vi "Autonomous Independent V.5.0.vi"() -> ()   [LabVIEW 2016]
doc: "This VI is called when autonomous begins, and will automatically be terminated when autonomous ends. You can carry out timed or sensor driven robot movement independently without needing to return to the caller."
uses:
  <vilib>/Rock Robotics/WPI/Camera/WPI_CameraImageSize.ctl
  <vilib>/Rock Robotics/WPI/ThirdParty/CanMotor/TalonSRX/WPI_CANTalonSRX_BrakeOverride.ctl
  <vilib>/Rock Robotics/WPI/Utilities/WPI_GetSetVariantRefNum.vi
  Robot Global Data V.5.0.vi
  <vilib>/Rock Robotics/Network Tables/NT Read String.vi
panel:
  out "Angle for Gyro":dbl
  out "image size":T1=enum."320x240"
  out "Height":dbl format="%#_13g"
  out "Width":dbl format="%#_13g"
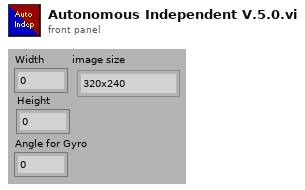
[diagram p1: front panel]
types:
  T1 = typedef "WPI_CameraImageSize.ctl" = enum16{"640x480", "320x240", "160x120", "Custom"}
  T2 = typedef "WPI_CANTalonSRX_BrakeOverride.ctl" = enum8{"No Override", "Override to Coast", "Override to Brake"}
  T3 = cluster{"Distance (ft)":dbl, "Score":dbl, "Normalized":cluster{"Center":cluster{dbl, dbl}, "Rectangle":cluster{"Numeric":dbl, "Numeric 2":dbl, "Numeric 3":dbl, "Numeric 5":dbl}}, "Pixels":cluster{"Center":cluster{dbl, dbl}, "Rectangle":cluster{"Numeric":dbl, "Numeric 2":dbl, "Numeric 3":dbl, "Numeric 5":dbl}}}
  T4 = cluster{"Center":cluster{dbl, dbl}, "Rectangle":cluster{"Numeric":dbl, "Numeric 2":dbl, "Numeric 3":dbl, "Numeric 5":dbl}}
  T5 = cluster{"Numeric":dbl, "Numeric 2":dbl, "Numeric 3":dbl, "Numeric 5":dbl}
  T6 = typedef "WPI_RobotDriveDevRef.ctl" = cluster{"DevStatus":errorcluster, "Motors[]":T7[], "Square Inputs":bool, "Max Output":dbl}
  T7 = typedef "WPI_MotorControlDeviceRef.ctl" = cluster{"DeviceStatus":errorcluster, "Type":T8, "PWM":cluster{"PWM Channel":T9, "DeadBand":T10}, "CAN":cluster{"Device Number":u8, "SetOutput VI Ref":variant, "GetOutput VI Ref":variant, "Enable VI Ref":variant, "Disable VI Ref":variant, "Data":variant}, "Invert":bool}
  T8 = typedef "WPI_MotorControlType.ctl" = enum16{"PWM", "CAN"}
  T9 = typedef "FPGA_DIOPWMChannel.ctl" = enum8{"PWM 0", "PWM 1", "PWM 2", "PWM 3", "PWM 4", "PWM 5", "PWM 6", "PWM 7", "PWM 8", "PWM 9", "PWM MXP 0", "PWM MXP 1", "PWM MXP 2", "PWM MXP 3", "PWM MXP 4", "PWM MXP 5", "PWM MXP 6", "PWM MXP 7", "PWM MXP 8", "PWM MXP 9", "Invalid"}
  T10 = typedef "WPI_PWMDeadband.ctl" = cluster{"Name":string, "maxPositivePwm":i32, "minPositivePwm":i32, "centerPwm":i32, "maxNegativePwm":i32, "minNegativePwm":i32, "angularRange":u16}
  T11 = typedef "WPI_CANTalonSRX_GlobalStatus.ctl" = cluster{"Applied Throttle":dbl, "Module Enabled":bool, "CAN Error":errorcluster, "Closed Loop Error":dbl, "Forward Limit Switch Closed":bool, "Reverse Limit Switch Closed":bool, "Sensor Position":dbl, "Sensor Velocity":dbl, "Current":dbl, "Sticky Fault - Over Temp":bool, "Sticky Fault - Under Voltage":bool, "Sticky Fault - Forward Limit":bool, "Sticky Fault - Reverse Limit":bool, "Sticky Fault - Forward Soft Limit":bool, "Sticky Fault - Reverse Soft Limit":bool, "Brake is Enabled":bool, "Encoder Position":dbl, "Encoder Velocity":dbl, "Encoder Index Count":dbl, "Encoder A Pin State":bool, "Encoder B Pin State":bool, "Encoder Index Pin State":bool, "Analog In":dbl, "Analog In Velocity":dbl, "Temperature (C)":dbl, "Battery Voltage":dbl, "Control 5 Is Supported":bool, "Current Profile Slot Select":dbl, "Pos Div 8":bool, "Vel Div 4":bool, "Pulse Width Position":i32, "Pulse Width Velocity":i32, "Pulse Width Rise To Rise (us)":i32, "Pulse Width Rise To Fall (us)":i32, "Mot Prof Active Is Under Run":bool, "Mot Prof Active Has Under Run":bool, "Mot Prof Active Is Last":bool, "Mot Prof Active Velocity Only":bool, "Mot Prof Active Is Valid":bool, "Mot Prof Buffer Is Full":bool, "Mot Prof Active Profile Slot Select":i32, "Mot Prof NextID":i32, "Mot Prof Count":i32, "Mot Prof Active Velocity":dbl, "Mot Prof Active Position":dbl, "Mot Prof Output Enable":i32}
  T12 = typedef "WPI_GyroDevRef.ctl" = cluster{"DevStatus":errorcluster, "Analog Channel":T13, "Offset":dbl, "Gain (VoltsPerDegree/Second)":dbl, "Gyro Type":enum16{"Analog", "XRS450"}, "Handle":i32, "SPI Bus":T14, "Device Found":bool, "Sample Rate":dbl, "Calibrate On Open":bool}
  T13 = typedef "FPGA_AIChannel.ctl" = enum8{"AI 0", "AI 1", "AI 2", "AI 3", "AI MXP 0", "AI MXP 1", "AI MXP 2", "AI MXP 3", "Invalid"}
  T14 = typedef "spi_bus.ctl" = enum16{"SPI On-Board, CS0", "SPI On-Board, CS1", "SPI On-Board, CS2", "SPI On-Board, CS3", "SPI MXP", "Invalid"}
  T15 = typedef "WPI_ServoDeviceRef.ctl" = cluster{"DeviceStatus":errorcluster, "PWM Channel":T9, "DeadBand":T10}
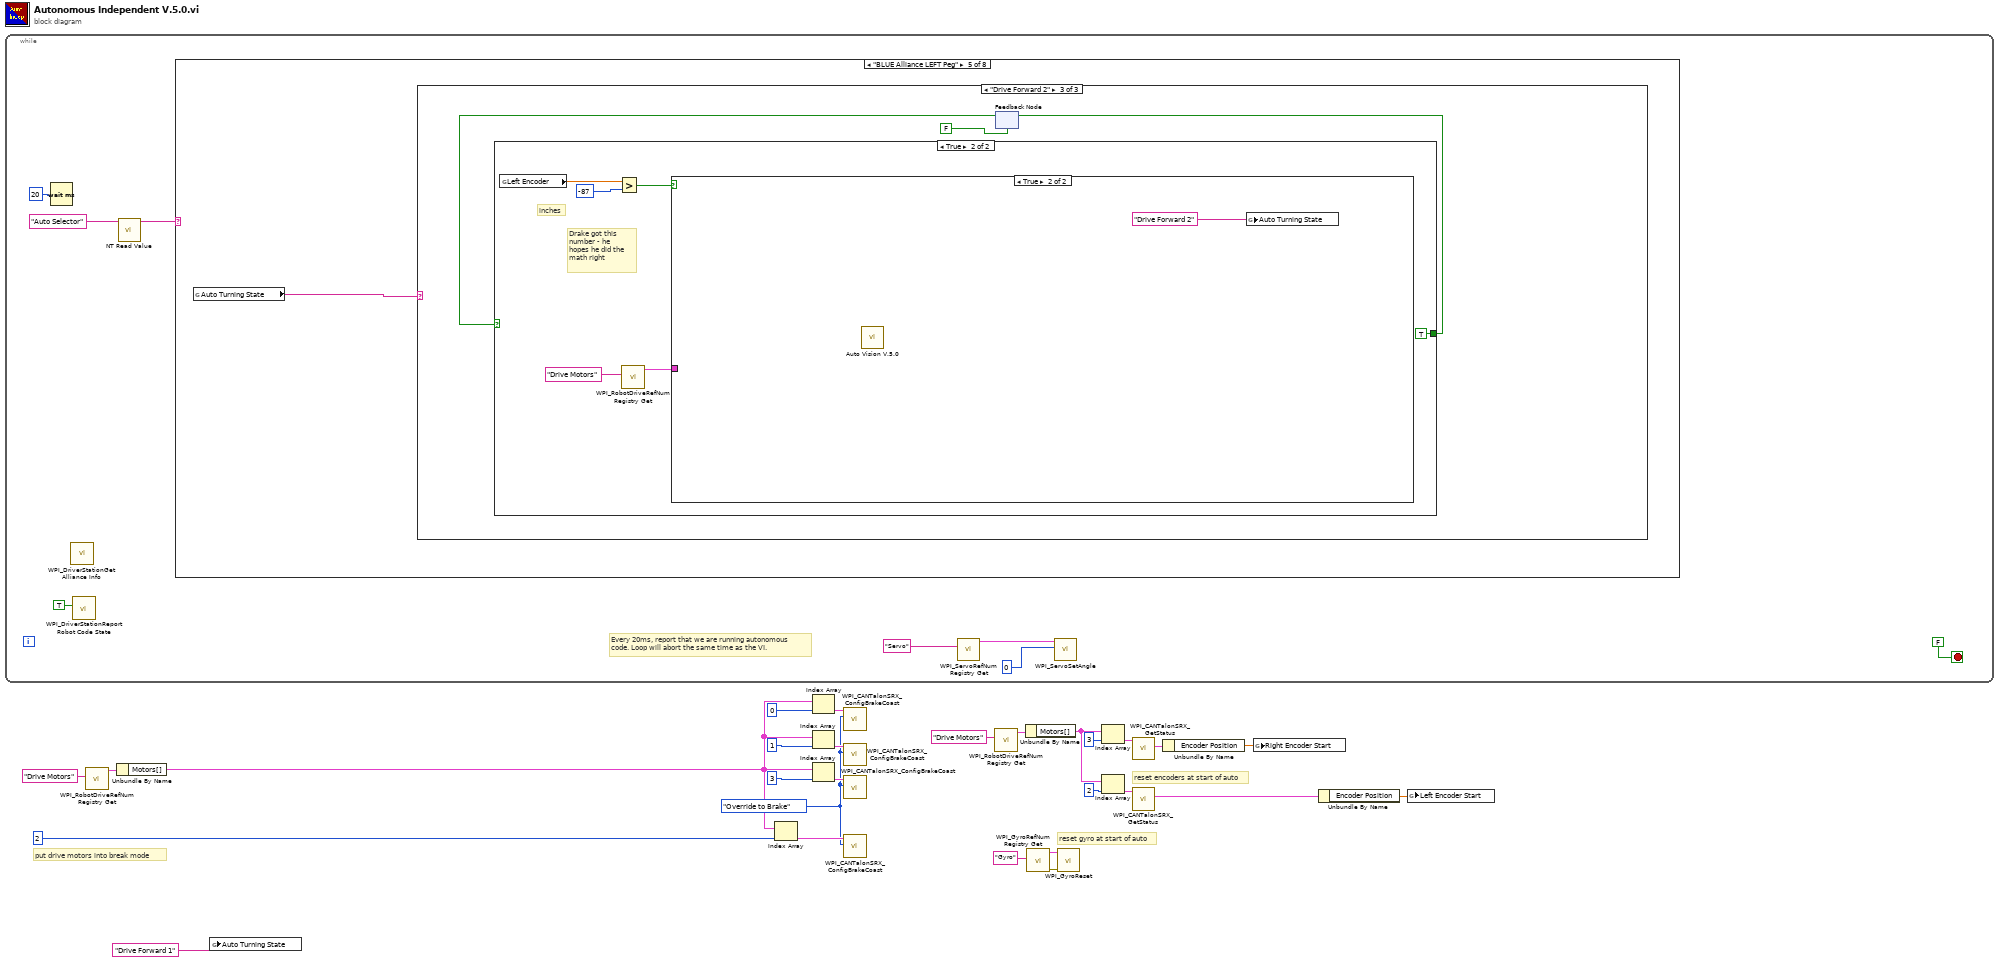
[diagram p0: block diagram]
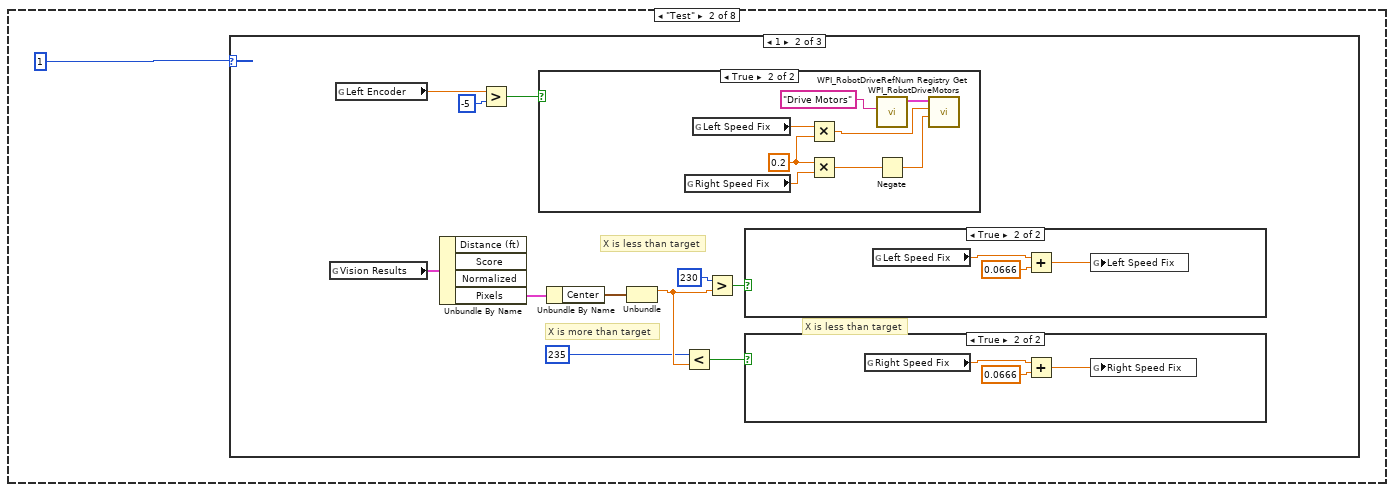
[diagram p3: hidden frame]
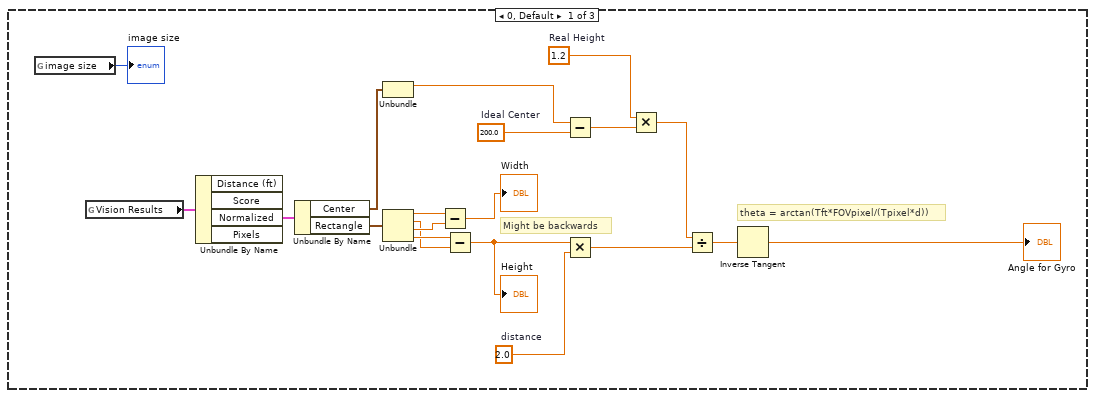
[diagram p4: hidden frame]
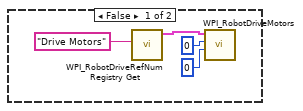
[diagram p5: hidden frame]
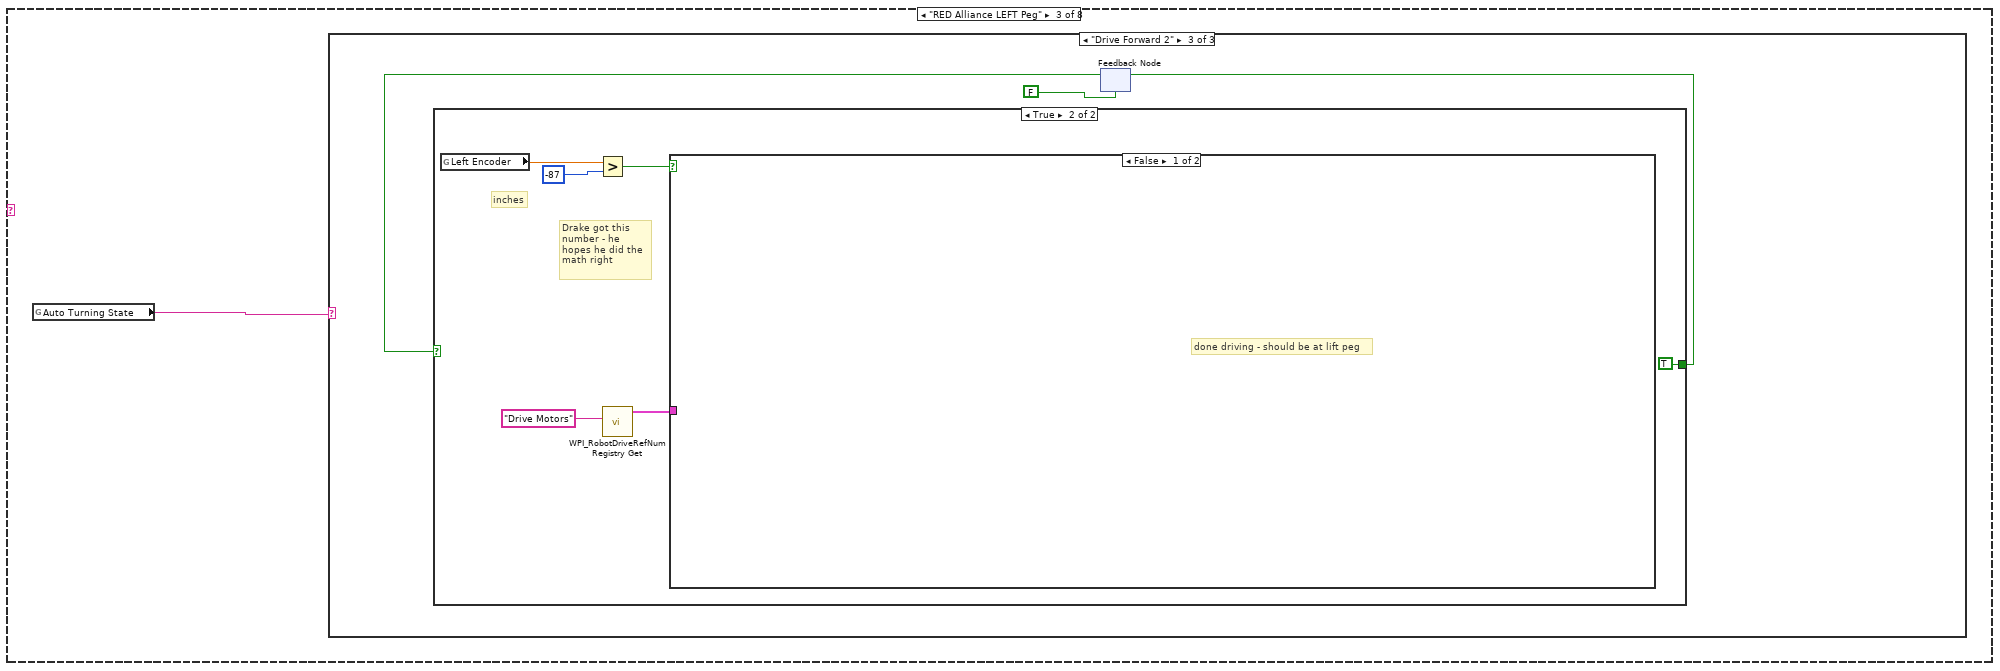
[diagram p9: hidden frame]
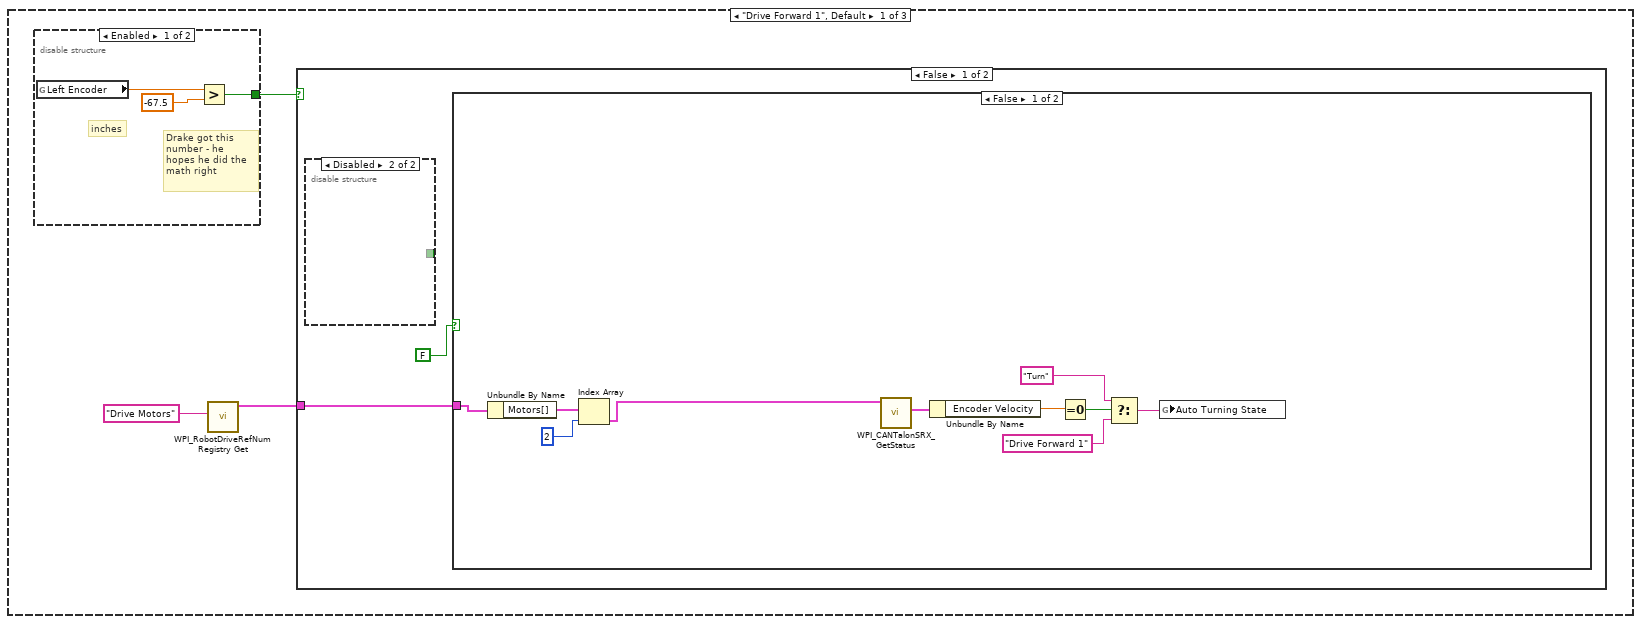
[diagram p10: hidden frame]
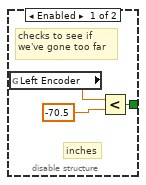
[diagram p12: hidden frame]
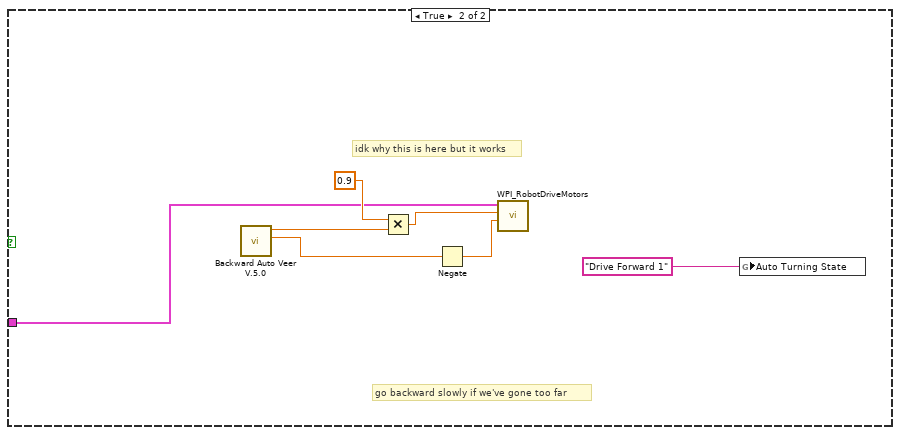
[diagram p13: hidden frame]
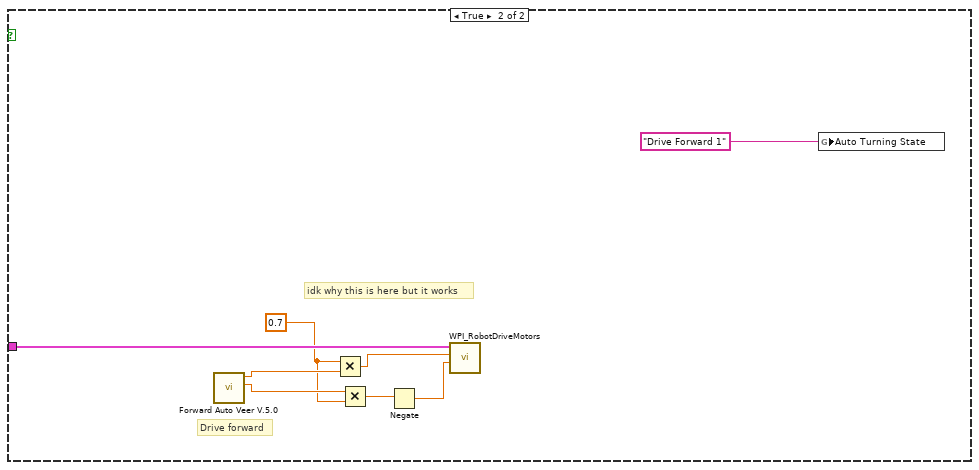
[diagram p14: hidden frame]
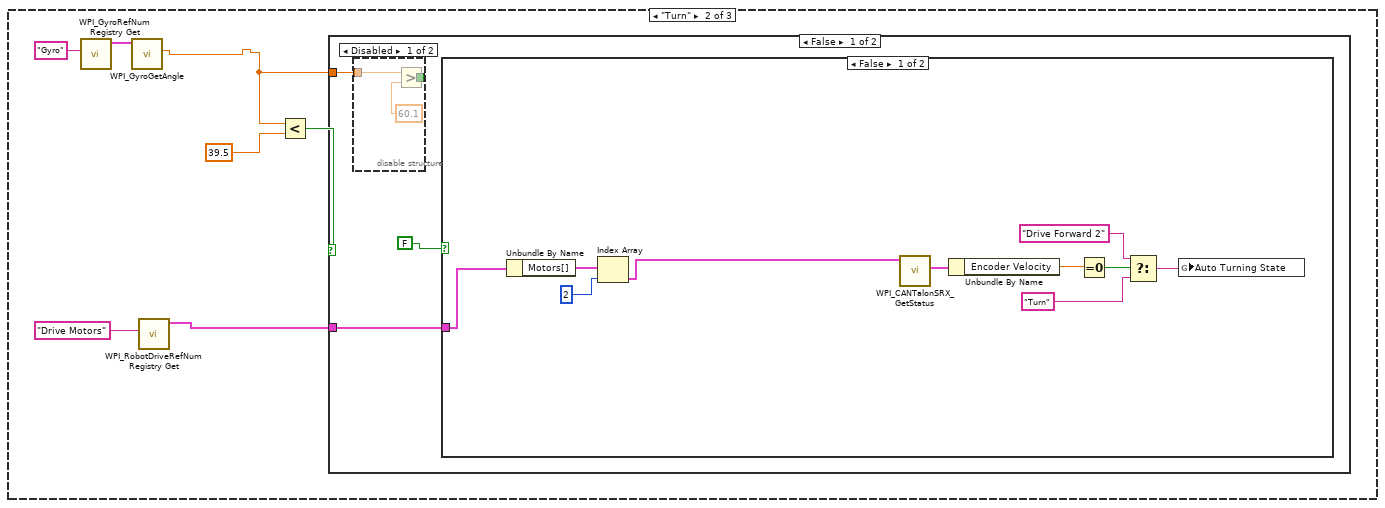
[diagram p15: hidden frame]
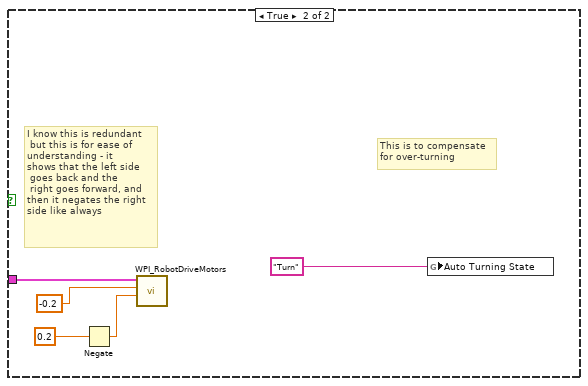
[diagram p17: hidden frame]
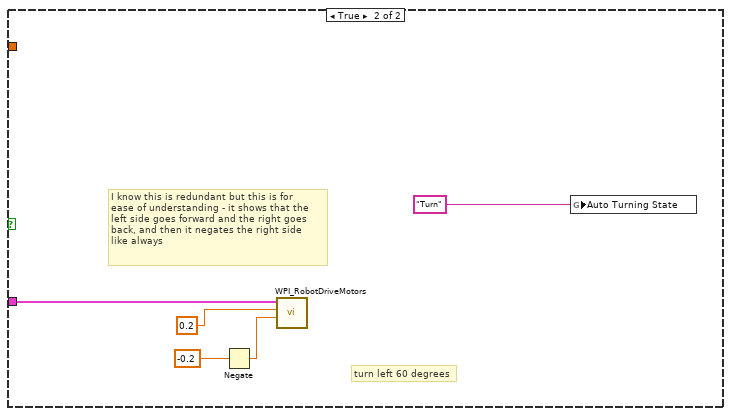
[diagram p18: hidden frame]
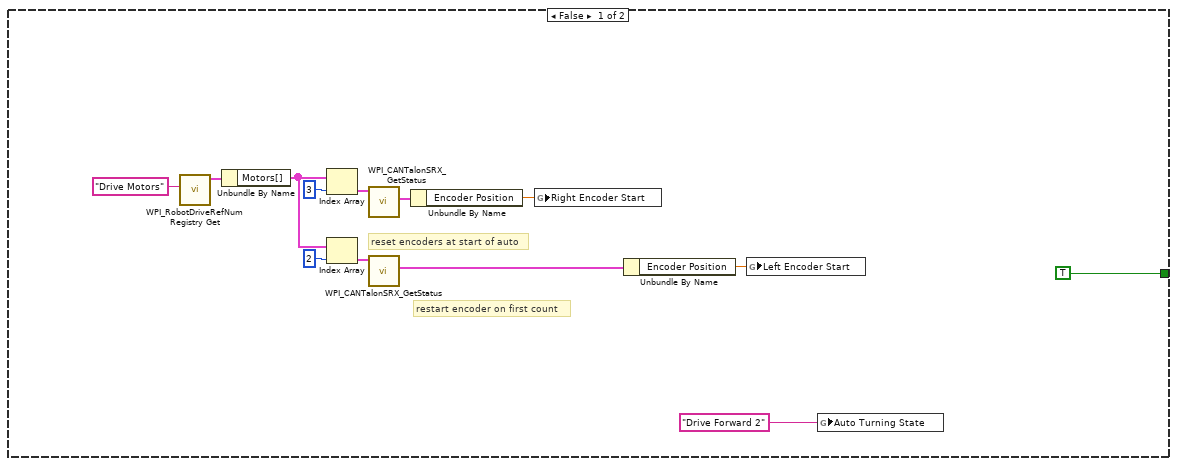
[diagram p19: hidden frame]
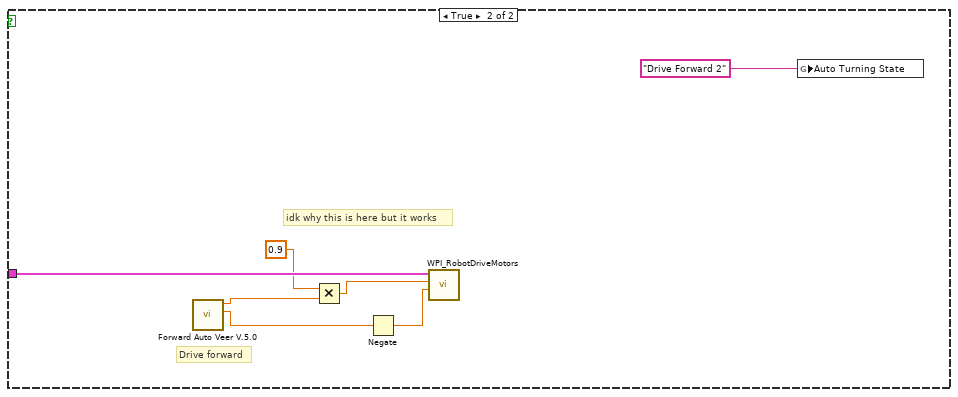
[diagram p20: hidden frame]
diagram:
  w5 = WPI_CANTalonSRX_BrakeOverride."Override to Brake" ("Brake / Coast Mode")
  # "put drive motors into break mode"
  # "reset gyro at start of auto"
  # "reset encoders at start of auto"
  n1 = while {
    stop <- FALSE stop-if-true
    # "Every 20ms, report that we are running autonomous\ncode. Loop will abort the same time as the VI."
    n2 = Wait (ms)(milliseconds to wait=u32 20) -> ()  [unwired: 1 out]
    n3 = call <vilib>:"WPI_DriverStationGet Alliance Info.vi"() -> ()  [unwired: 12 out]
    n4 = call <vilib>:"WPI_DriverStationReport Robot Code State.vi"("Autonomous"=TRUE) -> ()  [unwired: 10 in, 1 out]
    n5 = call-poly <vilib>:"NT Read Value.vi"("Name"="Auto Selector") -> ("String"=w34:string)  [unwired: 9 in, 1 out]
    n6 = case shown="\"BLUE Alliance LEFT Peg\"" w34 {
      frame Default {
        # "You can put your main auto here, or you can right-click on the case and make any\nother frame be the default case."
        # "This is the frame that will execute if no selection is made, or if it is not recognized"
      }
      frame "Test" {
        n7 = case shown="1" 1 {
          frame 0, Default {
            w39 = 200.0  # Ideal Center
            w44 = 2.0  # distance
            w49 = 1.2  # Real Height
            # "theta = arctan(Tft*FOVpixel/(Tpixel*d))"
            # "Might be backwards"
            n8 = global read "Robot Global Data V.5.0.vi" "image size"() -> (→"image size":T1)
            n9 = global read "Robot Global Data V.5.0.vi" "Vision Results"() -> (w56:T3)
            n10 = Unbundle By Name(w56) -> ("Normalized"=w55:T4)  [unwired: 3 out]
            n11 = Unbundle By Name(w55) -> ("Center"=w40:cluster{dbl, dbl}, "Rectangle"=w54:T5)
            n12 = Unbundle(w40) -> (w38:dbl)  [unwired: 1 out]
            n13 = Unbundle(w54) -> ("Numeric"=w53:dbl, "Numeric 2"=w42:dbl, "Numeric 3"=w52:dbl, "Numeric 5"=w43:dbl)
            n14 = Subtract(x=w53, y=w52) -> (x-y=→"Width":dbl)
            n15 = Subtract(x=w43, y=w42) -> (x-y=w41:dbl)
            "Height" <- w41
            n16 = Subtract(x=w38, y=w39) -> (x-y=w37:dbl)
            n17 = Multiply(x=w41, y=w44) -> (x*y=w46:dbl)
            n18 = Multiply(x=w49, y=w37) -> (x*y=w47:dbl)
            n19 = Divide(x=w47, y=w46) -> (x/y=w48:dbl)
            n20 = Inverse Tangent(1:w48) -> (0:→"Angle for Gyro":dbl)
          }
          frame 1 {
            # "X is less than target"
            # "X is more than target"
            # "X is less than target"
            n21 = global read "Robot Global Data V.5.0.vi" "Vision Results"() -> (w67:T3)
            n22 = global read "Robot Global Data V.5.0.vi" "Left Encoder"() -> (w57:dbl)
            n23 = Unbundle By Name(w67) -> ("Pixels"=w66:T4)  [unwired: 3 out]
            n24 = Greater?(x=w57, y=-5) -> (0:w59:bool)
            n25 = case shown="True" w59 {
              frame False {
                n26 = call <vilib>:"WPI_RobotDriveRefNum Registry Get.vi"("refnum name"="Drive Motors") -> ("RobotDriveDevRef"=w70:T6)  [unwired: 9 in, 1 out]
                n27 = call <vilib>:"WPI_RobotDriveMotors.vi"("RightSpeed"=0, "LeftSpeed"=0, "RobotDriveDevRef"=w70) -> ()  [unwired: 6 in, 3 out]
              }
              frame True {
                w77 = 0.2
                n28 = global read "Robot Global Data V.5.0.vi" "Right Speed Fix"() -> (w76:dbl)
                n29 = global read "Robot Global Data V.5.0.vi" "Left Speed Fix"() -> (w75:dbl)
                n30 = Multiply(x=w75, y=w77) -> (x*y=w74:dbl)
                n31 = Multiply(x=w77, y=w76) -> (x*y=w73:dbl)
                n32 = call <vilib>:"WPI_RobotDriveRefNum Registry Get.vi"("refnum name"="Drive Motors") -> ("RobotDriveDevRef"=w78:T6)  [unwired: 9 in, 1 out]
                n33 = Negate(x=w73) -> (-x=w72:dbl)
                n34 = call <vilib>:"WPI_RobotDriveMotors.vi"("RightSpeed"=w72, "LeftSpeed"=w74, "RobotDriveDevRef"=w78) -> ()  [unwired: 6 in, 3 out]
              }
            }
            n35 = Unbundle By Name(w66) -> ("Center"=w65:cluster{dbl, dbl})
            n36 = Unbundle(w65) -> (w64:dbl)  [unwired: 1 out]
            n37 = Less?(x=235, y=w64) -> (x < y?=w61:bool)
            n38 = Greater?(x=230, y=w64) -> (0:w62:bool)
            n39 = case shown="True" w62 {
              frame False {
              }
              frame True {
                n40 = global read "Robot Global Data V.5.0.vi" "Left Speed Fix"() -> (w85:dbl)
                n41 = Add(x=w85, y=0.0666) -> (x+y=w84:dbl)
                n42 = global write "Robot Global Data V.5.0.vi" "Left Speed Fix"(w84) -> ()
              }
            }
            n43 = case shown="True" w61 {
              frame False {
              }
              frame True {
                n44 = global read "Robot Global Data V.5.0.vi" "Right Speed Fix"() -> (w81:dbl)
                n45 = Add(x=w81, y=0.0666) -> (x+y=w82:dbl)
                n46 = global write "Robot Global Data V.5.0.vi" "Right Speed Fix"(w82) -> ()
              }
            }
          }
          frame 2 {
          }
        }
      }
      frame "RED Alliance LEFT Peg" {
        n47 = global read "Robot Global Data V.5.0.vi" "Auto Turning State"() -> (w86:string)
        n48 = case shown="\"Drive Forward 2\"" w86 {
          frame "Drive Forward 1", Default {
            n49 = disable-structure shown="Enabled" {
              disable-tunnel: [w90 _] -> w87
              frame Enabled {
                # "Drake got this\nnumber - he \nhopes he did the \nmath right"
                # "inches"
                n50 = global read "Robot Global Data V.5.0.vi" "Left Encoder"() -> (w92:dbl)
                n51 = Greater?(x=w92, y=-67.5) -> (0:w90:bool)
              }
              frame Disabled {
              }
            }
            n52 = call <vilib>:"WPI_RobotDriveRefNum Registry Get.vi"("refnum name"="Drive Motors") -> ("RobotDriveDevRef"=w88:T6)  [unwired: 9 in, 1 out]
            n53 = case shown="False" w87 {
              tunnel: w88 -> [w94 w122]
              frame False {
                n54 = disable-structure shown="Disabled" {
                  disable-tunnel: [w95 _] -> _
                  frame Enabled {
                    # "checks to see if \nwe've gone too far"
                    # "inches"
                    n55 = global read "Robot Global Data V.5.0.vi" "Left Encoder"() -> (w97:dbl)
                    n56 = Less?(x=w97, y=-70.5) -> (x < y?=w95:bool)
                  }
                  frame Disabled {
                  }
                }
                n57 = case shown="False" FALSE {
                  tunnel: w94 -> [w107 w109]
                  frame False {
                    n58 = Unbundle By Name(w107) -> ("Motors[]"=w106:T7[])
                    n59 = Index Array(array=w106, index=2) -> (element=w104:T7)
                    n60 = call <vilib>:"WPI_CANTalonSRX_GetStatus.vi"("CAN Talon SRX Ref"=w104) -> ("Talon SRX Status"=w103:T11)  [unwired: 8 in, 2 out]
                    n61 = Unbundle By Name(w103) -> ("Encoder Velocity"=w102:dbl)
                    n62 = Equal To 0?(x=w102) -> (x = 0?=w101:bool)
                    n63 = Select(t="Turn", s=w101, f="Drive Forward 1") -> (s? t:f=w98:string)
                    n64 = global write "Robot Global Data V.5.0.vi" "Auto Turning State"(w98) -> ()
                  }
                  frame True {
                    # "go backward slowly if we've gone too far"
                    # "idk why this is here but it works"
                    n65 = call "Backward Auto Veer V.5.0.vi"() -> ("Right"=w110:dbl, "Left"=w111:dbl)  [unwired: 10 in]
                    n66 = Multiply(x=0.9, y=w111) -> (x*y=w112:dbl)
                    n67 = Negate(x=w110) -> (-x=w114:dbl)
                    n68 = call <vilib>:"WPI_RobotDriveMotors.vi"("RightSpeed"=w114, "LeftSpeed"=w112, "RobotDriveDevRef"=w109) -> ()  [unwired: 6 in, 3 out]
                    n69 = global write "Robot Global Data V.5.0.vi" "Auto Turning State"("Drive Forward 1") -> ()
                  }
                }
              }
              frame True {
                w115 = 0.7
                # "idk why this is here but it works"
                # "Drive forward"
                n70 = call "Forward Auto Veer V.5.0.vi"() -> ("Right"=w116:dbl, "Left"=w120:dbl)  [unwired: 10 in]
                n71 = Multiply(x=w115, y=w120) -> (x*y=w119:dbl)
                n72 = Multiply(x=w116, y=w115) -> (x*y=w117:dbl)
                n73 = Negate(x=w117) -> (-x=w121:dbl)
                n74 = call <vilib>:"WPI_RobotDriveMotors.vi"("RightSpeed"=w121, "LeftSpeed"=w119, "RobotDriveDevRef"=w122) -> ()  [unwired: 6 in, 3 out]
                n75 = global write "Robot Global Data V.5.0.vi" "Auto Turning State"("Drive Forward 1") -> ()
              }
            }
          }
          frame "Turn" {
            n76 = call <vilib>:"WPI_GyroRefNum Registry Get.vi"("refnum name"="Gyro") -> ("GyroDevRef"=w128:T12)  [unwired: 9 in, 1 out]
            n77 = call <vilib>:"WPI_GyroGetAngle.vi"("GyroDevRef"=w128) -> ("Angle"=w123:dbl)  [unwired: 6 in, 4 out]
            n78 = call <vilib>:"WPI_RobotDriveRefNum Registry Get.vi"("refnum name"="Drive Motors") -> ("RobotDriveDevRef"=w124:T6)  [unwired: 9 in, 1 out]
            n79 = Less?(x=w123, y=39.5) -> (x < y?=w126:bool)
            n80 = case shown="False" w126 {
              tunnel: w124 -> [w131 w155]
              tunnel: w123 -> [w132 _]
              frame False {
                n81 = disable-structure shown="Disabled" {
                  disable-tunnel: w132 -> [w134 _]
                  disable-tunnel: [w133 _] -> _
                  frame Disabled {
                    n82 = Greater?(x=w134, y=60.1) -> (0:w133:bool)
                  }
                  frame Enabled {
                  }
                }
                n83 = case shown="False" FALSE {
                  tunnel: w131 -> [w136 w147]
                  frame False {
                    n84 = Unbundle By Name(w136) -> ("Motors[]"=w145:T7[])
                    n85 = Index Array(array=w145, index=2) -> (element=w143:T7)
                    n86 = call <vilib>:"WPI_CANTalonSRX_GetStatus.vi"("CAN Talon SRX Ref"=w143) -> ("Talon SRX Status"=w142:T11)  [unwired: 8 in, 2 out]
                    n87 = Unbundle By Name(w142) -> ("Encoder Velocity"=w141:dbl)
                    n88 = Equal To 0?(x=w141) -> (x = 0?=w140:bool)
                    n89 = Select(t="Drive Forward 2", s=w140, f="Turn") -> (s? t:f=w137:string)
                    n90 = global write "Robot Global Data V.5.0.vi" "Auto Turning State"(w137) -> ()
                  }
                  frame True {
                    # "This is to compensate\nfor over-turning"
                    # "I know this is redundant\n but this is for ease of \nunderstanding - it \nshows that the left side\n goes back and the\n right goes forward, and \nthen it negates the right \nside like always"
                    n91 = Negate(x=0.2) -> (-x=w148:dbl)
                    n92 = call <vilib>:"WPI_RobotDriveMotors.vi"("RightSpeed"=w148, "LeftSpeed"=-0.2, "RobotDriveDevRef"=w147) -> ()  [unwired: 6 in, 3 out]
                    n93 = global write "Robot Global Data V.5.0.vi" "Auto Turning State"("Turn") -> ()
                  }
                }
              }
              frame True {
                # "turn left 60 degrees"
                # "I know this is redundant but this is for \nease of understanding - it shows that the\nleft side goes forward and the right goes\nback, and then it negates the right side \nlike always"
                n94 = Negate(x=-0.2) -> (-x=w152:dbl)
                n95 = call <vilib>:"WPI_RobotDriveMotors.vi"("RightSpeed"=w152, "LeftSpeed"=0.2, "RobotDriveDevRef"=w155) -> ()  [unwired: 6 in, 3 out]
                n96 = global write "Robot Global Data V.5.0.vi" "Auto Turning State"("Turn") -> ()
              }
            }
          }
          frame "Drive Forward 2" {
            n97 = feedback #1(FALSE) -> (w156:bool)
            n98 = case shown="True" w156 {
              tunnel: [TRUE TRUE] -> w158
              frame False {
                # "restart encoder on first count"
                # "reset encoders at start of auto"
                n99 = call <vilib>:"WPI_RobotDriveRefNum Registry Get.vi"("refnum name"="Drive Motors") -> ("RobotDriveDevRef"=w169:T6)  [unwired: 9 in, 1 out]
                n100 = Unbundle By Name(w169) -> ("Motors[]"=w160:T7[])
                n101 = Index Array(array=w160, index=3) -> (element=w163:T7)
                n102 = Index Array(array=w160, index=2) -> (element=w167:T7)
                n103 = call <vilib>:"WPI_CANTalonSRX_GetStatus.vi"("CAN Talon SRX Ref"=w163) -> ("Talon SRX Status"=w162:T11)  [unwired: 8 in, 2 out]
                n104 = call <vilib>:"WPI_CANTalonSRX_GetStatus.vi"("CAN Talon SRX Ref"=w167) -> ("Talon SRX Status"=w166:T11)  [unwired: 8 in, 2 out]
                n105 = Unbundle By Name(w162) -> ("Encoder Position"=w161:dbl)
                n106 = global write "Robot Global Data V.5.0.vi" "Right Encoder Start"(w161) -> ()
                n107 = Unbundle By Name(w166) -> ("Encoder Position"=w165:dbl)
                n108 = global write "Robot Global Data V.5.0.vi" "Left Encoder Start"(w165) -> ()
                n109 = global write "Robot Global Data V.5.0.vi" "Auto Turning State"("Drive Forward 2") -> ()
              }
              frame True {
                # "Drake got this\nnumber - he \nhopes he did the \nmath right"
                # "inches"
                n110 = global read "Robot Global Data V.5.0.vi" "Left Encoder"() -> (w177:dbl)
                n111 = Greater?(x=w177, y=-87) -> (0:w175:bool)
                n112 = call <vilib>:"WPI_RobotDriveRefNum Registry Get.vi"("refnum name"="Drive Motors") -> ("RobotDriveDevRef"=w173:T6)  [unwired: 9 in, 1 out]
                n113 = case shown="False" w175 {
                  tunnel: w173 -> [_ w184]
                  frame False {
                    # "done driving - should be at lift peg"
                  }
                  frame True {
                    # "idk why this is here but it works"
                    # "Drive forward"
                    n114 = call "Forward Auto Veer V.5.0.vi"() -> ("Right"=w182:dbl, "Left"=w181:dbl)  [unwired: 10 in]
                    n115 = Multiply(x=0.9, y=w181) -> (x*y=w179:dbl)
                    n116 = Negate(x=w182) -> (-x=w183:dbl)
                    n117 = call <vilib>:"WPI_RobotDriveMotors.vi"("RightSpeed"=w183, "LeftSpeed"=w179, "RobotDriveDevRef"=w184) -> ()  [unwired: 6 in, 3 out]
                    n118 = global write "Robot Global Data V.5.0.vi" "Auto Turning State"("Drive Forward 2") -> ()
                  }
                }
              }
            }
            n119 = feedback-in #1(w158) -> ()
          }
        }
      }
      frame "RED Alliance RIGHT Peg" {
        n120 = global read "Robot Global Data V.5.0.vi" "Auto Turning State"() -> (w185:string)
        n121 = case shown="\"Drive Forward 1\", Default" w185 {
          frame "Drive Forward 1", Default {
            # "Drake got this\nnumber - he \nhopes he did the \nmath right"
            # "inches"
            n122 = global read "Robot Global Data V.5.0.vi" "Left Encoder"() -> (w190:dbl)
            n123 = Greater?(x=w190, y=-40) -> (0:w188:bool)
            n124 = call <vilib>:"WPI_RobotDriveRefNum Registry Get.vi"("refnum name"="Drive Motors") -> ("RobotDriveDevRef"=w186:T6)  [unwired: 9 in, 1 out]
            n125 = case shown="False" w188 {
              tunnel: w186 -> [w192 w219]
              frame False {
                n126 = disable-structure shown="Disabled" {
                  disable-tunnel: [w193 _] -> _
                  frame Disabled {
                    # "checks to see if \nwe've gone too far"
                    # "inches"
                    n127 = global read "Robot Global Data V.5.0.vi" "Left Encoder"() -> (w195:dbl)
                    n128 = Less?(x=w195, y=-56) -> (x < y?=w193:bool)
                  }
                  frame Enabled {
                  }
                }
                n129 = case shown="False" FALSE {
                  tunnel: w192 -> [w205 w207]
                  frame False {
                    n130 = Unbundle By Name(w205) -> ("Motors[]"=w204:T7[])
                    n131 = Index Array(array=w204, index=2) -> (element=w202:T7)
                    n132 = call <vilib>:"WPI_CANTalonSRX_GetStatus.vi"("CAN Talon SRX Ref"=w202) -> ("Talon SRX Status"=w201:T11)  [unwired: 8 in, 2 out]
                    n133 = Unbundle By Name(w201) -> ("Encoder Velocity"=w200:dbl)
                    n134 = Equal To 0?(x=w200) -> (x = 0?=w199:bool)
                    n135 = Select(t="Turn", s=w199, f="Drive Forward 1") -> (s? t:f=w196:string)
                    n136 = global write "Robot Global Data V.5.0.vi" "Auto Turning State"(w196) -> ()
                  }
                  frame True {
                    # "go backward slowly if we've gone too far"
                    # "idk why this is here but it works"
                    n137 = call "Backward Auto Veer V.5.0.vi"() -> ("Right"=w208:dbl, "Left"=w209:dbl)  [unwired: 10 in]
                    n138 = Multiply(x=0.9, y=w209) -> (x*y=w210:dbl)
                    n139 = Negate(x=w208) -> (-x=w212:dbl)
                    n140 = call <vilib>:"WPI_RobotDriveMotors.vi"("RightSpeed"=w212, "LeftSpeed"=w210, "RobotDriveDevRef"=w207) -> ()  [unwired: 6 in, 3 out]
                    n141 = global write "Robot Global Data V.5.0.vi" "Auto Turning State"("Drive Forward 1") -> ()
                  }
                }
              }
              frame True {
                # "idk why this is here but it works"
                # "Drive forward"
                n142 = call "Forward Auto Veer V.5.0.vi"() -> ("Right"=w217:dbl, "Left"=w216:dbl)  [unwired: 10 in]
                n143 = Multiply(x=0.9, y=w216) -> (x*y=w214:dbl)
                n144 = Negate(x=w217) -> (-x=w218:dbl)
                n145 = call <vilib>:"WPI_RobotDriveMotors.vi"("RightSpeed"=w218, "LeftSpeed"=w214, "RobotDriveDevRef"=w219) -> ()  [unwired: 6 in, 3 out]
                n146 = global write "Robot Global Data V.5.0.vi" "Auto Turning State"("Drive Forward 1") -> ()
              }
            }
          }
          frame "Turn" {
            n147 = call <vilib>:"WPI_GyroRefNum Registry Get.vi"("refnum name"="Gyro") -> ("GyroDevRef"=w225:T12)  [unwired: 9 in, 1 out]
            n148 = call <vilib>:"WPI_GyroGetAngle.vi"("GyroDevRef"=w225) -> ("Angle"=w222:dbl)  [unwired: 6 in, 4 out]
            n149 = call <vilib>:"WPI_RobotDriveRefNum Registry Get.vi"("refnum name"="Drive Motors") -> ("RobotDriveDevRef"=w220:T6)  [unwired: 9 in, 1 out]
            n150 = Greater?(x=w222, y=-39.5) -> (0:w223:bool)
            n151 = case shown="False" w223 {
              tunnel: w220 -> [w228 w252]
              tunnel: w222 -> [w229 _]
              frame False {
                n152 = disable-structure shown="Disabled" {
                  disable-tunnel: w229 -> [w231 _]
                  disable-tunnel: [w230 _] -> _
                  frame Disabled {
                    n153 = Less?(x=w231, y=-60.1) -> (x < y?=w230:bool)
                  }
                  frame Enabled {
                  }
                }
                n154 = case shown="False" FALSE {
                  tunnel: w228 -> [w233 w244]
                  frame False {
                    n155 = Unbundle By Name(w233) -> ("Motors[]"=w242:T7[])
                    n156 = Index Array(array=w242, index=2) -> (element=w240:T7)
                    n157 = call <vilib>:"WPI_CANTalonSRX_GetStatus.vi"("CAN Talon SRX Ref"=w240) -> ("Talon SRX Status"=w239:T11)  [unwired: 8 in, 2 out]
                    n158 = Unbundle By Name(w239) -> ("Encoder Velocity"=w238:dbl)
                    n159 = Equal To 0?(x=w238) -> (x = 0?=w237:bool)
                    n160 = Select(t="Drive Forward 2", s=w237, f="Turn") -> (s? t:f=w234:string)
                    n161 = global write "Robot Global Data V.5.0.vi" "Auto Turning State"(w234) -> ()
                  }
                  frame True {
                    # "This is to compensate\nfor over-turning"
                    # "I know this is redundant\n but this is for ease of \nunderstanding - it \nshows that the left side\n goes forward and the\n right goes back, and \nthen it negates the right \nside like always"
                    n162 = Negate(x=-0.3) -> (-x=w245:dbl)
                    n163 = call <vilib>:"WPI_RobotDriveMotors.vi"("RightSpeed"=w245, "LeftSpeed"=0.3, "RobotDriveDevRef"=w244) -> ()  [unwired: 6 in, 3 out]
                    n164 = global write "Robot Global Data V.5.0.vi" "Auto Turning State"("Turn") -> ()
                  }
                }
              }
              frame True {
                # "turn left 60 degrees"
                # "I know this is redundant but this is for \nease of understanding - it shows that the\nleft side goes back and the right goes\nforward, and then it negates the right side \nlike always"
                n165 = Negate(x=0.3) -> (-x=w249:dbl)
                n166 = call <vilib>:"WPI_RobotDriveMotors.vi"("RightSpeed"=w249, "LeftSpeed"=-0.3, "RobotDriveDevRef"=w252) -> ()  [unwired: 6 in, 3 out]
                n167 = global write "Robot Global Data V.5.0.vi" "Auto Turning State"("Turn") -> ()
              }
            }
          }
          frame "Drive Forward 2" {
            n168 = feedback #2(FALSE) -> (w253:bool)
            n169 = case shown="True" w253 {
              tunnel: [TRUE TRUE] -> w255
              frame False {
                # "restart encoder on first count"
                # "reset encoders at start of auto"
                n170 = call <vilib>:"WPI_RobotDriveRefNum Registry Get.vi"("refnum name"="Drive Motors") -> ("RobotDriveDevRef"=w266:T6)  [unwired: 9 in, 1 out]
                n171 = Unbundle By Name(w266) -> ("Motors[]"=w257:T7[])
                n172 = Index Array(array=w257, index=3) -> (element=w260:T7)
                n173 = Index Array(array=w257, index=2) -> (element=w264:T7)
                n174 = call <vilib>:"WPI_CANTalonSRX_GetStatus.vi"("CAN Talon SRX Ref"=w260) -> ("Talon SRX Status"=w259:T11)  [unwired: 8 in, 2 out]
                n175 = call <vilib>:"WPI_CANTalonSRX_GetStatus.vi"("CAN Talon SRX Ref"=w264) -> ("Talon SRX Status"=w263:T11)  [unwired: 8 in, 2 out]
                n176 = Unbundle By Name(w259) -> ("Encoder Position"=w258:dbl)
                n177 = global write "Robot Global Data V.5.0.vi" "Right Encoder Start"(w258) -> ()
                n178 = Unbundle By Name(w263) -> ("Encoder Position"=w262:dbl)
                n179 = global write "Robot Global Data V.5.0.vi" "Left Encoder Start"(w262) -> ()
                n180 = global write "Robot Global Data V.5.0.vi" "Auto Turning State"("Drive Forward 2") -> ()
              }
              frame True {
                # "Drake got this\nnumber - he \nhopes he did the \nmath right"
                # "inches"
                n181 = global read "Robot Global Data V.5.0.vi" "Left Encoder"() -> (w274:dbl)
                n182 = Greater?(x=w274, y=-87) -> (0:w272:bool)
                n183 = call <vilib>:"WPI_RobotDriveRefNum Registry Get.vi"("refnum name"="Drive Motors") -> ("RobotDriveDevRef"=w270:T6)  [unwired: 9 in, 1 out]
                n184 = case shown="True" w272 {
                  tunnel: w270 -> [_ w276]
                  frame False {
                    # "done driving - should be at lift peg"
                  }
                  frame True {
                    n185 = disable-structure shown="Disabled" {
                      disable-tunnel: w276 -> [w282 _]
                      frame Disabled {
                        # "idk why this is here but it works"
                        # "Drive forward"
                        n186 = call "Forward Auto Veer V.5.0.vi"() -> ("Right"=w280:dbl, "Left"=w279:dbl)  [unwired: 10 in]
                        n187 = Multiply(x=0.9, y=w279) -> (x*y=w277:dbl)
                        n188 = Negate(x=w280) -> (-x=w281:dbl)
                        n189 = call <vilib>:"WPI_RobotDriveMotors.vi"("RightSpeed"=w281, "LeftSpeed"=w277, "RobotDriveDevRef"=w282) -> ()  [unwired: 6 in, 3 out]
                      }
                      frame Enabled {
                      }
                    }
                    n190 = call "Auto Vision V.5.0.vi"() -> ()  [unwired: 12 in]
                    n191 = global write "Robot Global Data V.5.0.vi" "Auto Turning State"("Drive Forward 2") -> ()
                  }
                }
              }
            }
            n192 = feedback-in #2(w255) -> ()
          }
        }
      }
      frame "BLUE Alliance LEFT Peg" {
        n193 = global read "Robot Global Data V.5.0.vi" "Auto Turning State"() -> (w283:string)
        n194 = case shown="\"Drive Forward 2\"" w283 {
          frame "Drive Forward 1", Default {
            # "Drake got this\nnumber - he \nhopes he did the \nmath right"
            # "inches"
            n195 = global read "Robot Global Data V.5.0.vi" "Left Encoder"() -> (w288:dbl)
            n196 = Greater?(x=w288, y=-40) -> (0:w286:bool)
            n197 = call <vilib>:"WPI_RobotDriveRefNum Registry Get.vi"("refnum name"="Drive Motors") -> ("RobotDriveDevRef"=w284:T6)  [unwired: 9 in, 1 out]
            n198 = case shown="False" w286 {
              tunnel: w284 -> [w290 w317]
              frame False {
                n199 = disable-structure shown="Disabled" {
                  disable-tunnel: [w291 _] -> _
                  frame Disabled {
                    # "checks to see if \nwe've gone too far"
                    # "inches"
                    n200 = global read "Robot Global Data V.5.0.vi" "Left Encoder"() -> (w293:dbl)
                    n201 = Less?(x=w293, y=-56) -> (x < y?=w291:bool)
                  }
                  frame Enabled {
                  }
                }
                n202 = case shown="False" FALSE {
                  tunnel: w290 -> [w303 w305]
                  frame False {
                    n203 = Unbundle By Name(w303) -> ("Motors[]"=w302:T7[])
                    n204 = Index Array(array=w302, index=2) -> (element=w300:T7)
                    n205 = call <vilib>:"WPI_CANTalonSRX_GetStatus.vi"("CAN Talon SRX Ref"=w300) -> ("Talon SRX Status"=w299:T11)  [unwired: 8 in, 2 out]
                    n206 = Unbundle By Name(w299) -> ("Encoder Velocity"=w298:dbl)
                    n207 = Equal To 0?(x=w298) -> (x = 0?=w297:bool)
                    n208 = Select(t="Turn", s=w297, f="Drive Forward 1") -> (s? t:f=w294:string)
                    n209 = global write "Robot Global Data V.5.0.vi" "Auto Turning State"(w294) -> ()
                  }
                  frame True {
                    # "go backward slowly if we've gone too far"
                    # "idk why this is here but it works"
                    n210 = call "Backward Auto Veer V.5.0.vi"() -> ("Right"=w306:dbl, "Left"=w307:dbl)  [unwired: 10 in]
                    n211 = Multiply(x=0.9, y=w307) -> (x*y=w308:dbl)
                    n212 = Negate(x=w306) -> (-x=w310:dbl)
                    n213 = call <vilib>:"WPI_RobotDriveMotors.vi"("RightSpeed"=w310, "LeftSpeed"=w308, "RobotDriveDevRef"=w305) -> ()  [unwired: 6 in, 3 out]
                    n214 = global write "Robot Global Data V.5.0.vi" "Auto Turning State"("Drive Forward 1") -> ()
                  }
                }
              }
              frame True {
                # "idk why this is here but it works"
                # "Drive forward"
                n215 = call "Forward Auto Veer V.5.0.vi"() -> ("Right"=w315:dbl, "Left"=w314:dbl)  [unwired: 10 in]
                n216 = Multiply(x=0.9, y=w314) -> (x*y=w312:dbl)
                n217 = Negate(x=w315) -> (-x=w316:dbl)
                n218 = call <vilib>:"WPI_RobotDriveMotors.vi"("RightSpeed"=w316, "LeftSpeed"=w312, "RobotDriveDevRef"=w317) -> ()  [unwired: 6 in, 3 out]
                n219 = global write "Robot Global Data V.5.0.vi" "Auto Turning State"("Drive Forward 1") -> ()
              }
            }
          }
          frame "Turn" {
            n220 = call <vilib>:"WPI_GyroRefNum Registry Get.vi"("refnum name"="Gyro") -> ("GyroDevRef"=w323:T12)  [unwired: 9 in, 1 out]
            n221 = call <vilib>:"WPI_GyroGetAngle.vi"("GyroDevRef"=w323) -> ("Angle"=w320:dbl)  [unwired: 6 in, 4 out]
            n222 = call <vilib>:"WPI_RobotDriveRefNum Registry Get.vi"("refnum name"="Drive Motors") -> ("RobotDriveDevRef"=w318:T6)  [unwired: 9 in, 1 out]
            n223 = Less?(x=w320, y=39.5) -> (x < y?=w321:bool)
            n224 = case shown="True" w321 {
              tunnel: w318 -> [w326 w350]
              tunnel: w320 -> [w327 _]
              frame False {
                n225 = disable-structure shown="Disabled" {
                  disable-tunnel: w327 -> [w329 _]
                  disable-tunnel: [w328 _] -> _
                  frame Disabled {
                    n226 = Greater?(x=w329, y=60.1) -> (0:w328:bool)
                  }
                  frame Enabled {
                  }
                }
                n227 = case shown="True" FALSE {
                  tunnel: w326 -> [w331 w342]
                  frame False {
                    n228 = Unbundle By Name(w331) -> ("Motors[]"=w340:T7[])
                    n229 = Index Array(array=w340, index=2) -> (element=w338:T7)
                    n230 = call <vilib>:"WPI_CANTalonSRX_GetStatus.vi"("CAN Talon SRX Ref"=w338) -> ("Talon SRX Status"=w337:T11)  [unwired: 8 in, 2 out]
                    n231 = Unbundle By Name(w337) -> ("Encoder Velocity"=w336:dbl)
                    n232 = Equal To 0?(x=w336) -> (x = 0?=w335:bool)
                    n233 = Select(t="Drive Forward 2", s=w335, f="Turn") -> (s? t:f=w332:string)
                    n234 = global write "Robot Global Data V.5.0.vi" "Auto Turning State"(w332) -> ()
                  }
                  frame True {
                    # "This is to compensate\nfor over-turning"
                    # "I know this is redundant\n but this is for ease of \nunderstanding - it \nshows that the left side\n goes back and the\n right goes forward, and \nthen it negates the right \nside like always"
                    n235 = Negate(x=0.2) -> (-x=w343:dbl)
                    n236 = call <vilib>:"WPI_RobotDriveMotors.vi"("RightSpeed"=w343, "LeftSpeed"=-0.2, "RobotDriveDevRef"=w342) -> ()  [unwired: 6 in, 3 out]
                    n237 = global write "Robot Global Data V.5.0.vi" "Auto Turning State"("Turn") -> ()
                  }
                }
              }
              frame True {
                # "turn left 60 degrees"
                # "I know this is redundant but this is for \nease of understanding - it shows that the\nleft side goes forward and the right goes\nback, and then it negates the right side \nlike always"
                n238 = Negate(x=-0.2) -> (-x=w347:dbl)
                n239 = call <vilib>:"WPI_RobotDriveMotors.vi"("RightSpeed"=w347, "LeftSpeed"=0.2, "RobotDriveDevRef"=w350) -> ()  [unwired: 6 in, 3 out]
                n240 = global write "Robot Global Data V.5.0.vi" "Auto Turning State"("Turn") -> ()
              }
            }
          }
          frame "Drive Forward 2" {
            n241 = feedback #3(FALSE) -> (w351:bool)
            n242 = case shown="True" w351 {
              tunnel: [TRUE TRUE] -> w353
              frame False {
                # "restart encoder on first count"
                # "reset encoders at start of auto"
                n243 = call <vilib>:"WPI_RobotDriveRefNum Registry Get.vi"("refnum name"="Drive Motors") -> ("RobotDriveDevRef"=w364:T6)  [unwired: 9 in, 1 out]
                n244 = Unbundle By Name(w364) -> ("Motors[]"=w355:T7[])
                n245 = Index Array(array=w355, index=3) -> (element=w358:T7)
                n246 = Index Array(array=w355, index=2) -> (element=w362:T7)
                n247 = call <vilib>:"WPI_CANTalonSRX_GetStatus.vi"("CAN Talon SRX Ref"=w358) -> ("Talon SRX Status"=w357:T11)  [unwired: 8 in, 2 out]
                n248 = call <vilib>:"WPI_CANTalonSRX_GetStatus.vi"("CAN Talon SRX Ref"=w362) -> ("Talon SRX Status"=w361:T11)  [unwired: 8 in, 2 out]
                n249 = Unbundle By Name(w357) -> ("Encoder Position"=w356:dbl)
                n250 = global write "Robot Global Data V.5.0.vi" "Right Encoder Start"(w356) -> ()
                n251 = Unbundle By Name(w361) -> ("Encoder Position"=w360:dbl)
                n252 = global write "Robot Global Data V.5.0.vi" "Left Encoder Start"(w360) -> ()
                n253 = global write "Robot Global Data V.5.0.vi" "Auto Turning State"("Drive Forward 2") -> ()
              }
              frame True {
                # "Drake got this\nnumber - he \nhopes he did the \nmath right"
                # "inches"
                n254 = global read "Robot Global Data V.5.0.vi" "Left Encoder"() -> (w372:dbl)
                n255 = Greater?(x=w372, y=-87) -> (0:w370:bool)
                n256 = call <vilib>:"WPI_RobotDriveRefNum Registry Get.vi"("refnum name"="Drive Motors") -> ("RobotDriveDevRef"=w368:T6)  [unwired: 9 in, 1 out]
                n257 = case shown="True" w370 {
                  tunnel: w368 -> [_ _]
                  frame False {
                    # "done driving - should be at lift peg"
                  }
                  frame True {
                    n258 = call "Auto Vision V.5.0.vi"() -> ()  [unwired: 12 in]
                    n259 = global write "Robot Global Data V.5.0.vi" "Auto Turning State"("Drive Forward 2") -> ()
                  }
                }
              }
            }
            n260 = feedback-in #3(w353) -> ()
          }
        }
      }
      frame "BLUE Alliance RIGHT Peg" {
        n261 = global read "Robot Global Data V.5.0.vi" "Auto Turning State"() -> (w374:string)
        n262 = case shown="\"Drive Forward 1\", Default" w374 {
          frame "Drive Forward 1", Default {
            # "Drake got this\nnumber - he \nhopes he did the \nmath right"
            # "inches"
            n263 = global read "Robot Global Data V.5.0.vi" "Left Encoder"() -> (w379:dbl)
            n264 = Greater?(x=w379, y=-67.5) -> (0:w377:bool)
            n265 = call <vilib>:"WPI_RobotDriveRefNum Registry Get.vi"("refnum name"="Drive Motors") -> ("RobotDriveDevRef"=w375:T6)  [unwired: 9 in, 1 out]
            n266 = case shown="False" w377 {
              tunnel: w375 -> [w381 w408]
              frame False {
                n267 = disable-structure shown="Disabled" {
                  disable-tunnel: [w382 _] -> _
                  frame Disabled {
                    # "checks to see if \nwe've gone too far"
                    # "inches"
                    n268 = global read "Robot Global Data V.5.0.vi" "Left Encoder"() -> (w384:dbl)
                    n269 = Less?(x=w384, y=-69.5) -> (x < y?=w382:bool)
                  }
                  frame Enabled {
                  }
                }
                n270 = case shown="False" FALSE {
                  tunnel: w381 -> [w394 w396]
                  frame False {
                    n271 = Unbundle By Name(w394) -> ("Motors[]"=w393:T7[])
                    n272 = Index Array(array=w393, index=2) -> (element=w391:T7)
                    n273 = call <vilib>:"WPI_CANTalonSRX_GetStatus.vi"("CAN Talon SRX Ref"=w391) -> ("Talon SRX Status"=w390:T11)  [unwired: 8 in, 2 out]
                    n274 = Unbundle By Name(w390) -> ("Encoder Velocity"=w389:dbl)
                    n275 = Equal To 0?(x=w389) -> (x = 0?=w388:bool)
                    n276 = Select(t="Turn", s=w388, f="Drive Forward 1") -> (s? t:f=w385:string)
                    n277 = global write "Robot Global Data V.5.0.vi" "Auto Turning State"(w385) -> ()
                  }
                  frame True {
                    # "go backward slowly if we've gone too far"
                    # "idk why this is here but it works"
                    n278 = call "Backward Auto Veer V.5.0.vi"() -> ("Right"=w397:dbl, "Left"=w398:dbl)  [unwired: 10 in]
                    n279 = Multiply(x=0.9, y=w398) -> (x*y=w399:dbl)
                    n280 = Negate(x=w397) -> (-x=w401:dbl)
                    n281 = call <vilib>:"WPI_RobotDriveMotors.vi"("RightSpeed"=w401, "LeftSpeed"=w399, "RobotDriveDevRef"=w396) -> ()  [unwired: 6 in, 3 out]
                    n282 = global write "Robot Global Data V.5.0.vi" "Auto Turning State"("Drive Forward 1") -> ()
                  }
                }
              }
              frame True {
                # "idk why this is here but it works"
                # "Drive forward"
                n283 = call "Forward Auto Veer V.5.0.vi"() -> ("Right"=w406:dbl, "Left"=w405:dbl)  [unwired: 10 in]
                n284 = Multiply(x=0.9, y=w405) -> (x*y=w403:dbl)
                n285 = Negate(x=w406) -> (-x=w407:dbl)
                n286 = call <vilib>:"WPI_RobotDriveMotors.vi"("RightSpeed"=w407, "LeftSpeed"=w403, "RobotDriveDevRef"=w408) -> ()  [unwired: 6 in, 3 out]
                n287 = global write "Robot Global Data V.5.0.vi" "Auto Turning State"("Drive Forward 1") -> ()
              }
            }
          }
          frame "Turn" {
            n288 = call <vilib>:"WPI_GyroRefNum Registry Get.vi"("refnum name"="Gyro") -> ("GyroDevRef"=w414:T12)  [unwired: 9 in, 1 out]
            n289 = call <vilib>:"WPI_GyroGetAngle.vi"("GyroDevRef"=w414) -> ("Angle"=w411:dbl)  [unwired: 6 in, 4 out]
            n290 = call <vilib>:"WPI_RobotDriveRefNum Registry Get.vi"("refnum name"="Drive Motors") -> ("RobotDriveDevRef"=w409:T6)  [unwired: 9 in, 1 out]
            n291 = Greater?(x=w411, y=-59.9) -> (0:w412:bool)
            n292 = case shown="False" w412 {
              tunnel: w409 -> [w417 w441]
              tunnel: w411 -> [w418 _]
              frame False {
                n293 = disable-structure shown="Disabled" {
                  disable-tunnel: w418 -> [w420 _]
                  disable-tunnel: [w419 _] -> _
                  frame Disabled {
                    n294 = Less?(x=w420, y=-60.1) -> (x < y?=w419:bool)
                  }
                  frame Enabled {
                  }
                }
                n295 = case shown="True" FALSE {
                  tunnel: w417 -> [w422 w433]
                  frame False {
                    n296 = Unbundle By Name(w422) -> ("Motors[]"=w431:T7[])
                    n297 = Index Array(array=w431, index=2) -> (element=w429:T7)
                    n298 = call <vilib>:"WPI_CANTalonSRX_GetStatus.vi"("CAN Talon SRX Ref"=w429) -> ("Talon SRX Status"=w428:T11)  [unwired: 8 in, 2 out]
                    n299 = Unbundle By Name(w428) -> ("Encoder Velocity"=w427:dbl)
                    n300 = Equal To 0?(x=w427) -> (x = 0?=w426:bool)
                    n301 = Select(t="Drive Forward 2", s=w426, f="Turn") -> (s? t:f=w423:string)
                    n302 = global write "Robot Global Data V.5.0.vi" "Auto Turning State"(w423) -> ()
                  }
                  frame True {
                    # "This is to compensate\nfor over-turning"
                    # "I know this is redundant\n but this is for ease of \nunderstanding - it \nshows that the left side\n goes forward and the\n right goes back, and \nthen it negates the right \nside like always"
                    n303 = Negate(x=-0.2) -> (-x=w434:dbl)
                    n304 = call <vilib>:"WPI_RobotDriveMotors.vi"("RightSpeed"=w434, "LeftSpeed"=0.2, "RobotDriveDevRef"=w433) -> ()  [unwired: 6 in, 3 out]
                    n305 = global write "Robot Global Data V.5.0.vi" "Auto Turning State"("Turn") -> ()
                  }
                }
              }
              frame True {
                # "turn left 60 degrees"
                # "I know this is redundant but this is for \nease of understanding - it shows that the\nleft side goes back and the right goes\nforward, and then it negates the right side \nlike always"
                n306 = Negate(x=0.2) -> (-x=w438:dbl)
                n307 = call <vilib>:"WPI_RobotDriveMotors.vi"("RightSpeed"=w438, "LeftSpeed"=-0.2, "RobotDriveDevRef"=w441) -> ()  [unwired: 6 in, 3 out]
                n308 = global write "Robot Global Data V.5.0.vi" "Auto Turning State"("Turn") -> ()
              }
            }
          }
          frame "Drive Forward 2" {
            n309 = feedback #4(FALSE) -> (w442:bool)
            n310 = case shown="True" w442 {
              tunnel: [TRUE TRUE] -> w444
              frame False {
                # "restart encoder on first count"
                # "reset encoders at start of auto"
                n311 = call <vilib>:"WPI_RobotDriveRefNum Registry Get.vi"("refnum name"="Drive Motors") -> ("RobotDriveDevRef"=w455:T6)  [unwired: 9 in, 1 out]
                n312 = Unbundle By Name(w455) -> ("Motors[]"=w446:T7[])
                n313 = Index Array(array=w446, index=3) -> (element=w449:T7)
                n314 = Index Array(array=w446, index=2) -> (element=w453:T7)
                n315 = call <vilib>:"WPI_CANTalonSRX_GetStatus.vi"("CAN Talon SRX Ref"=w449) -> ("Talon SRX Status"=w448:T11)  [unwired: 8 in, 2 out]
                n316 = call <vilib>:"WPI_CANTalonSRX_GetStatus.vi"("CAN Talon SRX Ref"=w453) -> ("Talon SRX Status"=w452:T11)  [unwired: 8 in, 2 out]
                n317 = Unbundle By Name(w448) -> ("Encoder Position"=w447:dbl)
                n318 = global write "Robot Global Data V.5.0.vi" "Right Encoder Start"(w447) -> ()
                n319 = Unbundle By Name(w452) -> ("Encoder Position"=w451:dbl)
                n320 = global write "Robot Global Data V.5.0.vi" "Left Encoder Start"(w451) -> ()
                n321 = global write "Robot Global Data V.5.0.vi" "Auto Turning State"("Drive Forward 2") -> ()
              }
              frame True {
                # "Drake got this\nnumber - he \nhopes he did the \nmath right"
                # "inches"
                n322 = global read "Robot Global Data V.5.0.vi" "Left Encoder"() -> (w463:dbl)
                n323 = Greater?(x=w463, y=-87) -> (0:w461:bool)
                n324 = call <vilib>:"WPI_RobotDriveRefNum Registry Get.vi"("refnum name"="Drive Motors") -> ("RobotDriveDevRef"=w459:T6)  [unwired: 9 in, 1 out]
                n325 = case shown="False" w461 {
                  tunnel: w459 -> [_ w470]
                  frame False {
                    # "done driving - should be at lift peg"
                  }
                  frame True {
                    # "idk why this is here but it works"
                    # "Drive forward"
                    n326 = call "Forward Auto Veer V.5.0.vi"() -> ("Right"=w468:dbl, "Left"=w467:dbl)  [unwired: 10 in]
                    n327 = Multiply(x=0.9, y=w467) -> (x*y=w465:dbl)
                    n328 = Negate(x=w468) -> (-x=w469:dbl)
                    n329 = call <vilib>:"WPI_RobotDriveMotors.vi"("RightSpeed"=w469, "LeftSpeed"=w465, "RobotDriveDevRef"=w470) -> ()  [unwired: 6 in, 3 out]
                    n330 = global write "Robot Global Data V.5.0.vi" "Auto Turning State"("Drive Forward 2") -> ()
                  }
                }
              }
            }
            n331 = feedback-in #4(w444) -> ()
          }
        }
      }
      frame "MIDDLE Peg" {
        # "inches to\ndrive"
        n332 = global read "Robot Global Data V.5.0.vi" "Left Encoder"() -> (w471:dbl)
        n333 = Greater?(x=w471, y=-67.0) -> (0:w472:bool)
        n334 = call <vilib>:"WPI_RobotDriveRefNum Registry Get.vi"("refnum name"="Drive Motors") -> ("RobotDriveDevRef"=w473:T6)  [unwired: 9 in, 1 out]
        n335 = case shown="True" w472 {
          tunnel: w473 -> [_ w484]
          frame False {
          }
          frame True {
            w476 = 0.7
            # "idk why this is here but\nit works"
            n336 = call "Forward Auto Veer V.5.0.vi"() -> ("Right"=w478:dbl, "Left"=w480:dbl)  [unwired: 10 in]
            n337 = Multiply(x=w480, y=w476) -> (x*y=w479:dbl)
            n338 = Multiply(x=w476, y=w478) -> (x*y=w477:dbl)
            n339 = Negate(x=w477) -> (-x=w483:dbl)
            n340 = Multiply(x=0.9, y=w479) -> (x*y=w482:dbl)
            n341 = call <vilib>:"WPI_RobotDriveMotors.vi"("RightSpeed"=w483, "LeftSpeed"=w482, "RobotDriveDevRef"=w484) -> ()  [unwired: 6 in, 3 out]
          }
        }
      }
      frame "Baseline" {
        # "inches to drive"
        n342 = global read "Robot Global Data V.5.0.vi" "Left Encoder"() -> (w486:dbl)
        n343 = Greater?(x=w486, y=-80.0) -> (0:w485:bool)
        n344 = call <vilib>:"WPI_RobotDriveRefNum Registry Get.vi"("refnum name"="Drive Motors") -> ("RobotDriveDevRef"=w488:T6)  [unwired: 9 in, 1 out]
        n345 = case shown="True" w485 {
          tunnel: w488 -> [_ w495]
          frame False {
          }
          frame True {
            n346 = call "Forward Auto Veer V.5.0.vi"() -> ("Right"=w490:dbl, "Left"=w491:dbl)  [unwired: 10 in]
            n347 = Negate(x=w490) -> (-x=w494:dbl)
            n348 = Multiply(x=0.9, y=w491) -> (x*y=w493:dbl)
            n349 = call <vilib>:"WPI_RobotDriveMotors.vi"("RightSpeed"=w494, "LeftSpeed"=w493, "RobotDriveDevRef"=w495) -> ()  [unwired: 6 in, 3 out]
          }
        }
      }
    }
    n350 = call <vilib>:"WPI_ServoRefNum Registry Get.vi"("refnum name"="Servo") -> ("ServoDeviceRef"=w29:T15)  [unwired: 9 in, 1 out]
    n351 = call <vilib>:"WPI_ServoSetAngle.vi"("Angle"=0, "ServoDeviceRef"=w29) -> ()  [unwired: 8 in, 2 out]
  }
  n352 = call <vilib>:"WPI_RobotDriveRefNum Registry Get.vi"("refnum name"="Drive Motors") -> ("RobotDriveDevRef"=w15:T6)  [unwired: 9 in, 1 out]
  n353 = Unbundle By Name(w15) -> ("Motors[]"=w10:T7[])
  n354 = global write "Robot Global Data V.5.0.vi" "Auto Turning State"("Drive Forward 1") -> ()
  n355 = Index Array(array=w10, index=2) -> (element=w7:T7)
  n356 = Index Array(array=w10, index=0) -> (element=w9:T7)
  n357 = Index Array(array=w10, index=1) -> (element=w8:T7)
  n358 = Index Array(array=w10, index=3) -> (element=w6:T7)
  n359 = call <vilib>:"WPI_CANTalonSRX_ConfigBrakeCoast.vi"("Brake / Coast Mode"=w5, "CAN Talon SRX Ref"=w9) -> ()  [unwired: 8 in, 2 out]
  n360 = call <vilib>:"WPI_CANTalonSRX_ConfigBrakeCoast.vi"("Brake / Coast Mode"=w5, "CAN Talon SRX Ref"=w8) -> ()  [unwired: 8 in, 2 out]
  n361 = call <vilib>:"WPI_CANTalonSRX_ConfigBrakeCoast.vi"("Brake / Coast Mode"=w5, "CAN Talon SRX Ref"=w6) -> ()  [unwired: 8 in, 2 out]
  n362 = call <vilib>:"WPI_CANTalonSRX_ConfigBrakeCoast.vi"("Brake / Coast Mode"=w5, "CAN Talon SRX Ref"=w7) -> ()  [unwired: 8 in, 2 out]
  n363 = call <vilib>:"WPI_RobotDriveRefNum Registry Get.vi"("refnum name"="Drive Motors") -> ("RobotDriveDevRef"=w26:T6)  [unwired: 9 in, 1 out]
  n364 = Unbundle By Name(w26) -> ("Motors[]"=w17:T7[])
  n365 = call <vilib>:"WPI_GyroRefNum Registry Get.vi"("refnum name"="Gyro") -> ("error out"=w2:errorcluster, "GyroDevRef"=w3:T12)  [unwired: 9 in]
  n366 = call <vilib>:"WPI_GyroReset.vi"("error in"=w2, "GyroDevRef"=w3) -> ()  [unwired: 8 in, 2 out]
  n367 = Index Array(array=w17, index=3) -> (element=w20:T7)
  n368 = Index Array(array=w17, index=2) -> (element=w24:T7)
  n369 = call <vilib>:"WPI_CANTalonSRX_GetStatus.vi"("CAN Talon SRX Ref"=w20) -> ("Talon SRX Status"=w19:T11)  [unwired: 8 in, 2 out]
  n370 = call <vilib>:"WPI_CANTalonSRX_GetStatus.vi"("CAN Talon SRX Ref"=w24) -> ("Talon SRX Status"=w23:T11)  [unwired: 8 in, 2 out]
  n371 = Unbundle By Name(w19) -> ("Encoder Position"=w18:dbl)
  n372 = global write "Robot Global Data V.5.0.vi" "Right Encoder Start"(w18) -> ()
  n373 = Unbundle By Name(w23) -> ("Encoder Position"=w22:dbl)
  n374 = global write "Robot Global Data V.5.0.vi" "Left Encoder Start"(w22) -> ()
